vi "Tight Window.vi"() -> ()   [LabVIEW 2015]
uses:
  <vilib>/Utility/miscctls.llb/LVPointTypeDef.ctl
panel:
  in  "Tight Window Button":bool
  in  "stop":bool
  in  "VI":path
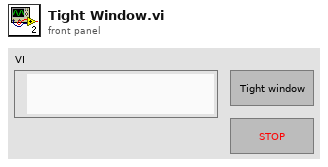
[diagram p1: front panel]
types:
  T1 = typedef "LVPointTypeDef.ctl" = cluster{"Horizontal":i16, "Vertical":i16}
  T2 = typedef "LVRectTypeDef.ctl" = cluster{"Left":i16, "Top":i16, "Right":i16, "Bottom":i16}
  T3 = typedef "LVBoundsTypeDef.ctl" = cluster{"Width":u32, "Height":u32}
  T4 = typedef "LVPositionTypeDef.ctl" = cluster{"Left":i32, "Top":i32}
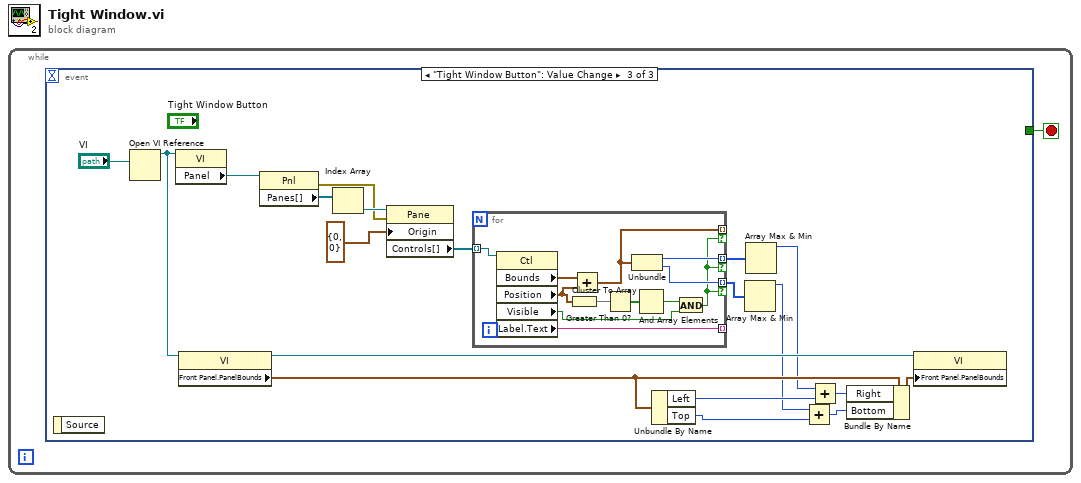
[diagram p0: block diagram]
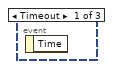
[diagram p2: hidden frame]
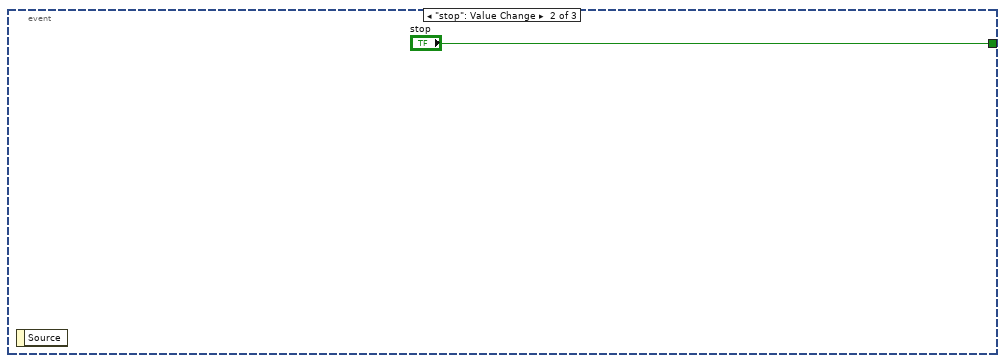
[diagram p3: hidden frame]
diagram:
  n1 = while {
    stop <- w1 stop-if-true
    n2 = event shown="[2] \"Tight Window Button\": Value Change" {
      selector: _ -> [_ _ _]
      dyn-events: _ -> [_ _ _]
      timeout: _ -> [_ _ _]
      tunnel: [_ "stop" _] -> w1
      event Timeout {
        n3 = event-data() -> ()  [unwired: 1 in, 1 out]
      }
      event "stop": Value Change {
        n4 = event-data() -> ()  [unwired: 1 in, 1 out]
      }
      event "Tight Window Button": Value Change {
        n5 = event-data() -> ()  [unwired: 1 in, 1 out]
        n6 = Open VI Reference(vi path="VI") -> (vi reference=w15:refnum<vi>)  [unwired: 5 in, 1 out]
        n7 = property class="VI"(reference=w15) -> ("Panel"=w16:refnum<vi>)  [unwired: 1 in, 2 out]
        n8 = property class="VI"(reference=w15) -> (reference out=w14:refnum<vi>, "Front Panel.PanelBounds"=w9:T2)  [unwired: 1 in, 1 out]
        n9 = property class="Pnl"(reference=w16) -> (error out=w18:errorcluster, "Panes[]"=w20:refnum<vi>[])  [unwired: 1 in, 1 out]
        n10 = Index Array(array=w20) -> (element=w19:refnum<vi>)  [unwired: 1 in]
        n11 = property class="Pane"(reference=w19, error in=w18, "Origin"=T1 {"Horizontal"=0, "Vertical"=0}) -> ("Controls[]"=w13:refnum<vi>[])  [unwired: 2 out]
        n12 = for {
          tunnel: w13 -> [w33] mode=indexing
          tunnel: [w25] -> w10 mode=indexing if=w23
          tunnel: [w26] -> w11 mode=indexing if=w23
          tunnel: [w24] -> _ mode=indexing if=w23
          tunnel: [w22] -> _ mode=indexing
          n13 = property class="Ctl"(reference=w33) -> ("Bounds"=w32:T3, "Position"=w31:T4, "Visible"=w27:bool, "Label.Text"=w22:string)  [unwired: 1 in, 2 out]
          n14 = Cluster To Array(cluster=w31) -> (array=w30:i32[])
          n15 = Add(x=w32, y=w31) -> (x+y=w24:T3)
          n16 = Greater Than 0?(x=w30) -> (x > 0?=w29:bool[])
          n17 = Unbundle(w24) -> ("Width"=w26:u32, "Height"=w25:u32)
          n18 = And Array Elements(Boolean array=w29) -> (logical AND=w28:bool)
          n19 = And(x=w28, y=w27) -> (x .and. y?=w23:bool)
        }
        n20 = Unbundle By Name(w9) -> ("Left"=w8:i16, "Top"=w5:i16)
        n21 = Array Max & Min(array=w10) -> (max value=w4:u32)  [unwired: 3 out]
        n22 = Array Max & Min(array=w11) -> (max value=w7:u32)  [unwired: 3 out]
        n23 = Add(x=w4, y=w5) -> (x+y=w3:u32)
        n24 = Add(x=w7, y=w8) -> (x+y=w6:u32)
        n25 = Bundle By Name(cluster=w9, "Right"=w6, "Bottom"=w3) -> (w12:T2)
        n26 = property class="VI"(reference=w14, "Front Panel.PanelBounds"=w12) -> ()  [unwired: 1 in, 2 out]
      }
    }
  }
